vi "TestExec.Result Option, Set Enable_Disabel Color.vi"(10 "Result Sel":refnum<vi>) -> ()   [LabVIEW 2018]
uses:
  TestExec.Result Option Selector.ctl
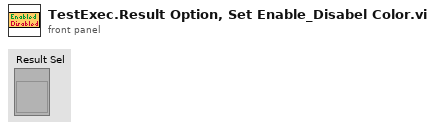
[diagram p1: front panel]
types:
  T1 = typedef "TestExec.Result Option Selector.ctl" = u16
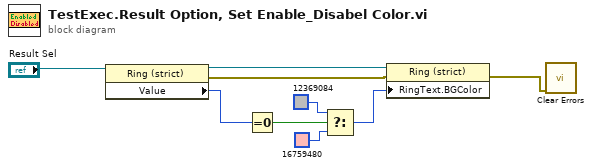
[diagram p0: block diagram]
diagram:
  n1 = property class="Ring (strict)"(reference="Result Sel") -> (reference out=w8:refnum<vi>, error out=w4:errorcluster, "Value"=w9:T1)  [unwired: 1 in]
  n2 = Equal To 0?(x=w9) -> (x = 0?=w3:bool)
  n3 = Select(t=u32 12369084, s=w3, f=u32 16759480) -> (s? t:f=w7:u32)
  n4 = property class="Ring (strict)"(reference=w8, error in=w4, "RingText.BGColor"=w7) -> (error out=w2:errorcluster)  [unwired: 1 out]
  n5 = call <vilib>:"Clear Errors.vi"("error in (no error)"=w2) -> ()  [unwired: 5 in, 2 out]
